vi "Control_ReadJoystick2.vi"() -> (4 "Up":bool, 6 "Down":bool, 8 "Left":bool, 10 "Right":bool, 15 "Button":bool)   [LabVIEW 2018]
uses:
  <vilib>/rvi/eio/common/nirviEmuTemplateMethod_errors.vi
  <vilib>/eio/EIONode/EIONode.xnode
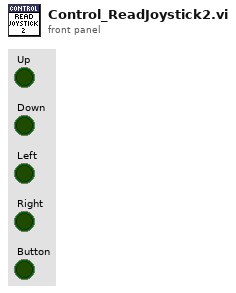
[diagram p1: front panel]
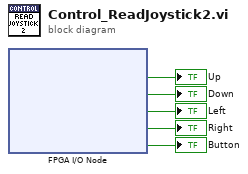
[diagram p0: block diagram]
diagram:
  n1 = xnode "FPGA I/O Node"() -> ("ConnectorA/DIO5"=→"Up":bool, "ConnectorA/DIO6"=→"Down":bool, "ConnectorA/DIO7"=→"Left":bool, "ConnectorA/DIO8"=→"Right":bool, "ConnectorA/DIO9"=→"Button":bool)  [unwired: 5 in, 5 out]
